vi "Ctor.vi"(8 "error in (no error)":errorcluster) -> (0 "error out":errorcluster, 3 "DeviceManager out":refnum<class "DeviceManager.lvclass">)   [LabVIEW 2020, in "PicoG-Core.lvlib" / "DeviceManager.lvclass"]
uses:
  DeviceManager.lvclass
  DeployResource/DeployResource.lvclass
  Device/Device.lvclass
  DeviceManager.lvclass/DeviceManager.ctl
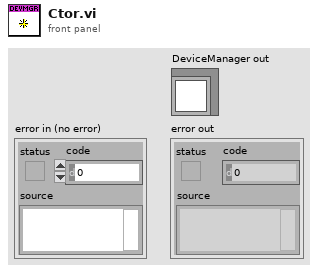
[diagram p1: front panel]
types:
  T1 = map{refnum<class "DeployResource.lvclass">, refnum<class "Device.lvclass">}
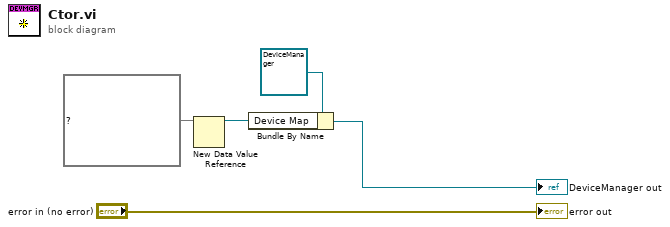
[diagram p0: block diagram]
diagram:
  n1 = New Data Value Reference(data value=T1 {} ("map")) -> (data value reference=w1:refnum<data-value>)  [unwired: 1 in, 1 out]
  n2 = Bundle By Name(cluster=refnum<class "DeviceManager.lvclass"> refnum ("DeviceManager in"), "Device Map"=w1) -> (→"DeviceManager out":refnum<class "DeviceManager.lvclass">)
  "error out" <- "error in (no error)"
